vi "PWM_testVI.vi"() -> ()   [LabVIEW 2019]
panel:
  in  "PWM positions":dbl[](array[numeric])=[4.5, 3.4, 4.6, 8.4]
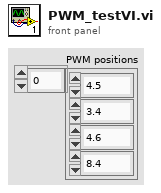
[diagram p1: front panel]
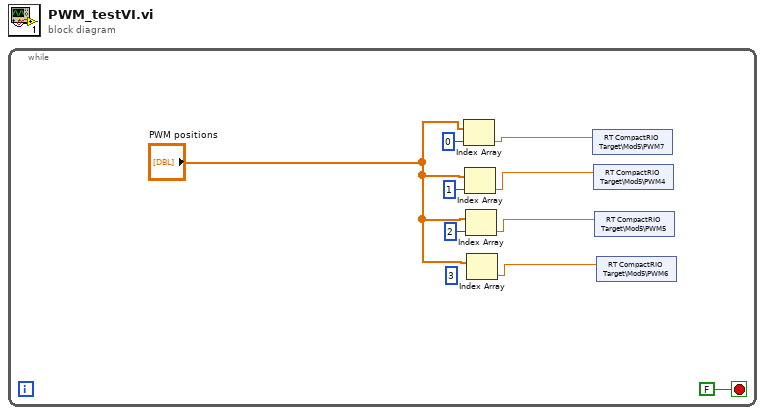
[diagram p0: block diagram]
diagram:
  n1 = while {
    stop <- FALSE stop-if-true
    (unwired) 3 ("index")
    n2 = Index Array(array="PWM positions", index=0) -> (element=w4:dbl)
    n3 = Index Array(array="PWM positions", index=1) -> (element=w3:dbl)
    n4 = Index Array(array="PWM positions", index=2) -> (element=w8:dbl)
    n5 = Index Array(array="PWM positions") -> (element=w9:dbl)  [unwired: 1 in]
    n6 = shared-variable "RT CompactRIO Target\\Mod5\\PWM7"(w4) -> ()  [unwired: 1 in, 1 out]
    n7 = shared-variable "RT CompactRIO Target\\Mod5\\PWM4"(w3) -> ()  [unwired: 1 in, 1 out]
    n8 = shared-variable "RT CompactRIO Target\\Mod5\\PWM5"(w8) -> ()  [unwired: 1 in, 1 out]
    n9 = shared-variable "RT CompactRIO Target\\Mod5\\PWM6"(w9) -> ()  [unwired: 1 in, 1 out]
  }
